vi "getKeyFormatAndValChkRes.vi"(7 "entryName":string, 8 "error in":errorcluster, 9 "arg":string, 10 "sec":string, 11 "Tree Refnum in":refnum<vi>) -> (0 "error out":errorcluster, 1 "Check result":string="√", 2 "entryFormat":string, 3 "Tree Refnum out":refnum<vi>)   [LabVIEW 2010]
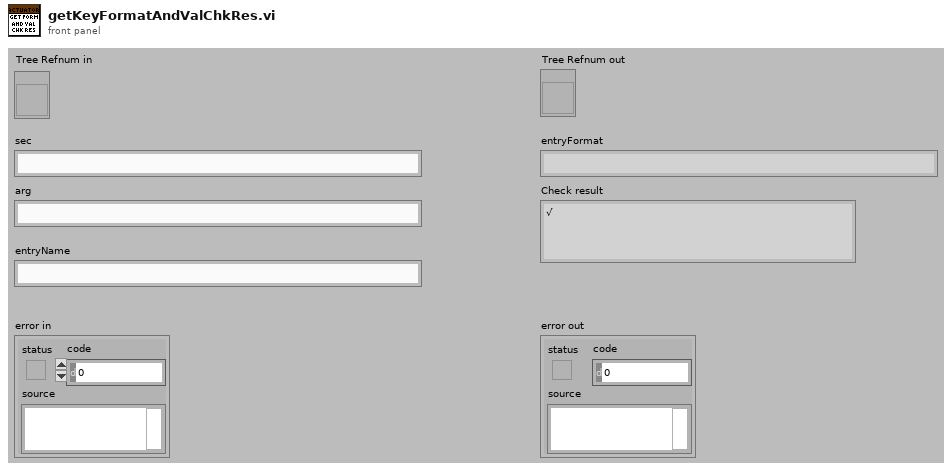
[diagram p1: front panel]
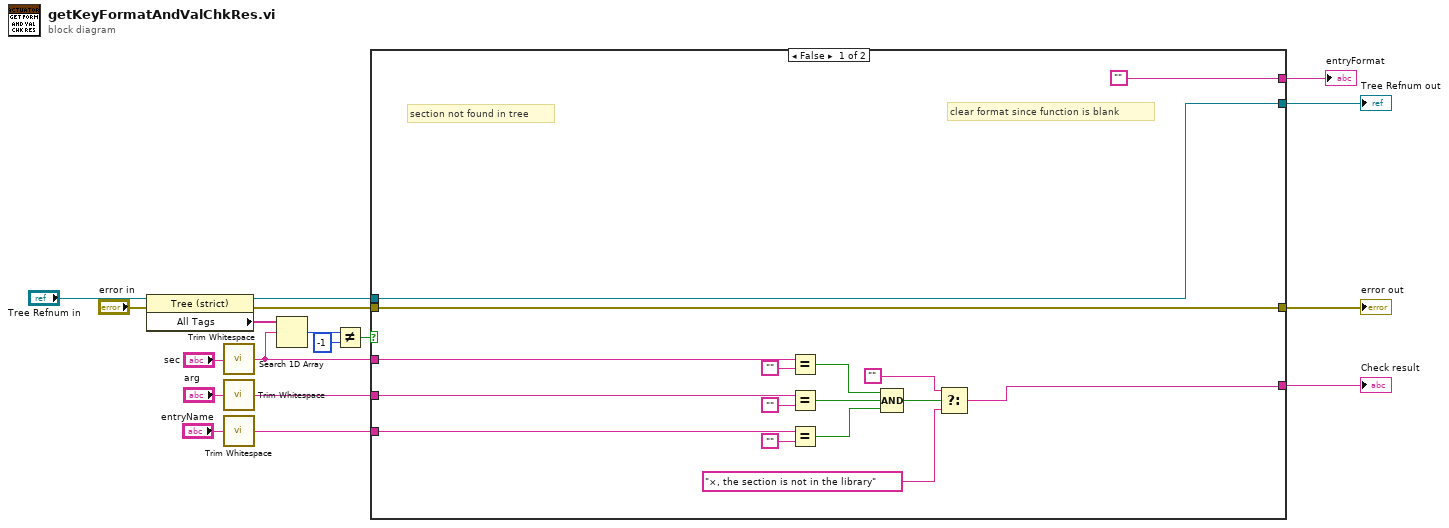
[diagram p0: block diagram]
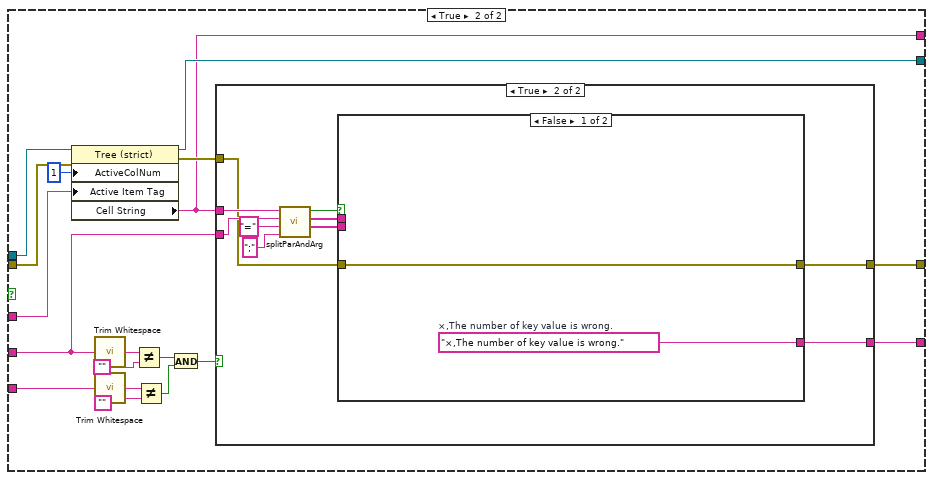
[diagram p2: hidden frame]
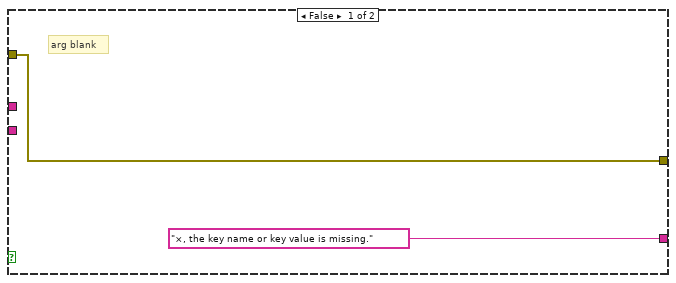
[diagram p3: hidden frame]
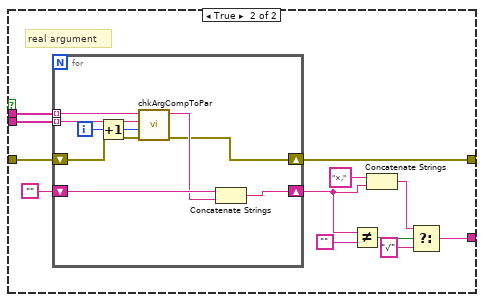
[diagram p4: hidden frame]
diagram:
  n1 = property on="Property Node" class="Tree (strict)"(reference="Tree Refnum in", error in="error in") -> (reference out=w12:refnum<vi>, error out=w5:errorcluster, "All Tags"=w15:string[])
  n2 = call <vilib>:"Trim Whitespace.vi"("string"="sec") -> ("trimmed string"=w4:string)  [unwired: 1 in]
  n3 = call <vilib>:"Trim Whitespace.vi"("string"="arg") -> ("trimmed string"=w7:string)  [unwired: 1 in]
  n4 = call <vilib>:"Trim Whitespace.vi"("string"="entryName") -> ("trimmed string"=w1:string)  [unwired: 1 in]
  n5 = Search 1D Array(1D array=w15, element=w4) -> (index of element=w14:i32)  [unwired: 1 in]
  n6 = Not Equal?(x=w14, y=-1) -> (x != y?=w18:bool)
  n7 = case shown="False" w18 {
    tunnel: w7 -> [w32 w48]
    tunnel: [w28 w52] -> w17
    tunnel: [w27 w51] -> w16
    tunnel: w12 -> [w34 w46]
    tunnel: [w34 w42] -> w11
    tunnel: w5 -> [w27 w45]
    tunnel: w4 -> [w25 w44]
    tunnel: ["" w41] -> w3
    tunnel: w1 -> [w23 w40]
    frame False {
      # "clear format since function is blank"
      # "section not found in tree"
      n8 = Equal?(x=w25, y="") -> (x = y?=w21:bool)
      n9 = Equal?(x=w32, y="") -> (x = y?=w20:bool)
      n10 = Equal?(x=w23, y="") -> (x = y?=w19:bool)
      n11 = Compound Arithmetic op=AND(w21, w20, w19) -> (w31:bool)
      n12 = Select(t="", s=w31, f="×, the section is not in the library") -> (s? t:f=w28:string)
    }
    frame True {
      n13 = property class="Tree (strict)"(reference=w46, error in=w45, "ActiveColNum"=1 ("Active Cell:Active Column Number"), "Active Item Tag"=w44) -> (reference out=w42:refnum<vi>, error out=w43:errorcluster, "Cell String"=w41:string)
      n14 = call <vilib>:"Trim Whitespace.vi"("string"=w48) -> ("trimmed string"=w50:string)  [unwired: 1 in]
      n15 = call <vilib>:"Trim Whitespace.vi"("string"=w40) -> ("trimmed string"=w39:string)  [unwired: 1 in]
      n16 = Not Equal?(x=w50, y="") -> (x != y?=w37:bool)
      n17 = Not Equal?(x=w39, y="") -> (x != y?=w36:bool)
      n18 = And(x=w37, y=w36) -> (x .and. y?=w35:bool)
      n19 = case shown="True" w35 {
        tunnel: w41 -> [_ w62]
        tunnel: w48 -> [_ w61]
        tunnel: w43 -> [w54 w55]
        tunnel: ["×, the key name or key value is missing." w64] -> w52
        tunnel: [w54 w63] -> w51
        frame False {
          # "arg blank"
        }
        frame True {
          n20 = call "splitParAndArg.vi"("paraEndMark"=";" ("regular expression"), "paraStartMark"="=" ("regular expression"), "allArguments"=w61, "allParameters"=w62) -> ("argArray"=w58:string[], "paraArray"=w57:string[], "sameNum?"=w56:bool)  [unwired: 5 in]
          n21 = case shown="False" w56 {
            tunnel: w57 -> [_ w78]
            tunnel: w58 -> [_ w77]
            tunnel: [w66 w72] -> w64
            tunnel: w55 -> [w65 w71]
            tunnel: [w65 w70] -> w63
            frame False {
              w66 = "×,The number of key value is wrong."  # ×,The number of key value is wrong.
            }
            frame True {
              # "real argument"
              n22 = for {
                tunnel: w78 -> [w87] mode=indexing
                tunnel: w77 -> [w86] mode=indexing
                shift-right: [w79] -> w68
                shift-left: "" -> [w82]
                shift-right: [w80] -> w70
                shift-left: w71 -> [w83]
                i -> [w85]
                n23 = Increment(x=w85) -> (x+1=w84:i32)
                n24 = call "chkArgCompToPar.vi"("error in"=w83, "argSN"=w84, "arg"=w86, "par"=w87) -> ("error out"=w80:errorcluster, "judgement"=w81:string)  [unwired: 6 in]
                n25 = Concatenate Strings(w82, w81) -> (w79:string)
              }
              n26 = Not Equal?(x=w68, y="") -> (x != y?=w74:bool)
              n27 = Concatenate Strings("×,", w68) -> (w67:string)
              n28 = Select(t=w67, s=w74, f="√") -> (s? t:f=w72:string)
            }
          }
        }
      }
    }
  }
  "Check result" <- w17
  "error out" <- w16
  "Tree Refnum out" <- w11
  "entryFormat" <- w3
